vi "Global Sensors.vi"() -> ()   [LabVIEW 2019]
panel:
  out "Switch_ToShooter":bool
  in  "ColorSensor":string
  out "Switch_Conveyor":bool
  in  "Ultrasonic_Shooter":bool
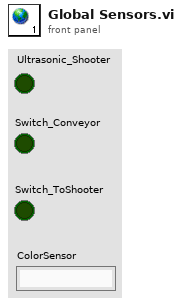
[diagram p1: front panel]
diagram:
